vi "zmq_req LabVIEW client.vi"() -> ()   [LabVIEW 2019]
uses:
  <vilib>/addons/zeromq/socket_type.ctl
  <vilib>/addons/zeromq/zmq_context.lvclass
  <vilib>/addons/zeromq/zeromq.lvlib
  <vilib>/addons/zeromq/zmq_socket.lvclass
  erx-demo/eRX 802.15.4/Performance measure context.ctl
panel:
  out "data":string
  out "Measures out":T1 {"Total samples" format="%#_6p"; "Elapsed time" format="%#_6p"; "Samples per second" format="%#_6p"; "Time per sample" format="%#_6p"; "Packets per second" format="%#_6p"; "Last samples per second" format="%#_6p"}
  out "error out":errorcluster
  in  "Stop 2":bool
  in  "Stop":bool
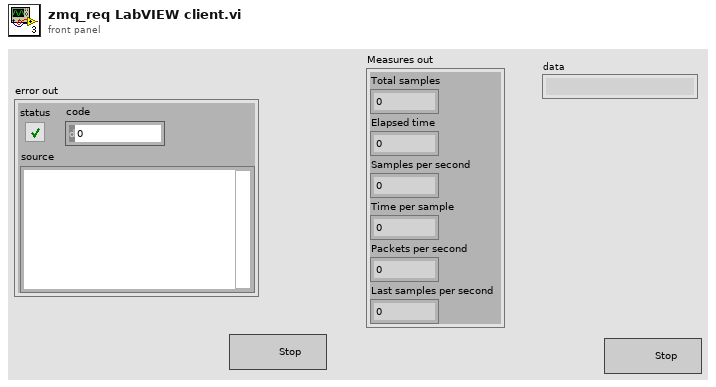
[diagram p1: front panel]
types:
  T1 = cluster{"Total samples":dbl, "Elapsed time":dbl, "Samples per second":dbl, "Time per sample":dbl, "Packets per second":dbl, "Last samples per second":dbl}
  T2 = typedef "zeromq.lvlib/socket_type.ctl" = enum8{"ZMQ_PAIR", "ZMQ_PUB", "ZMQ_SUB", "ZMQ_REQ", "ZMQ_REP", "ZMQ_DEALER", "ZMQ_ROUTER", "ZMQ_PULL", "ZMQ_PUSH", "ZMQ_XPUB", "ZMQ_XSUB"}
  T3 = typedef "Performance measure context.ctl" = cluster{"Seconds decayed":dbl, "Samples decayed":dbl, "Packet count":dbl, "Samples count":dbl, "Timestamp":dbl, "Start time":dbl}
  T4 = enum16{"Standard", "Buffered", "CRLF", "Immediate"}
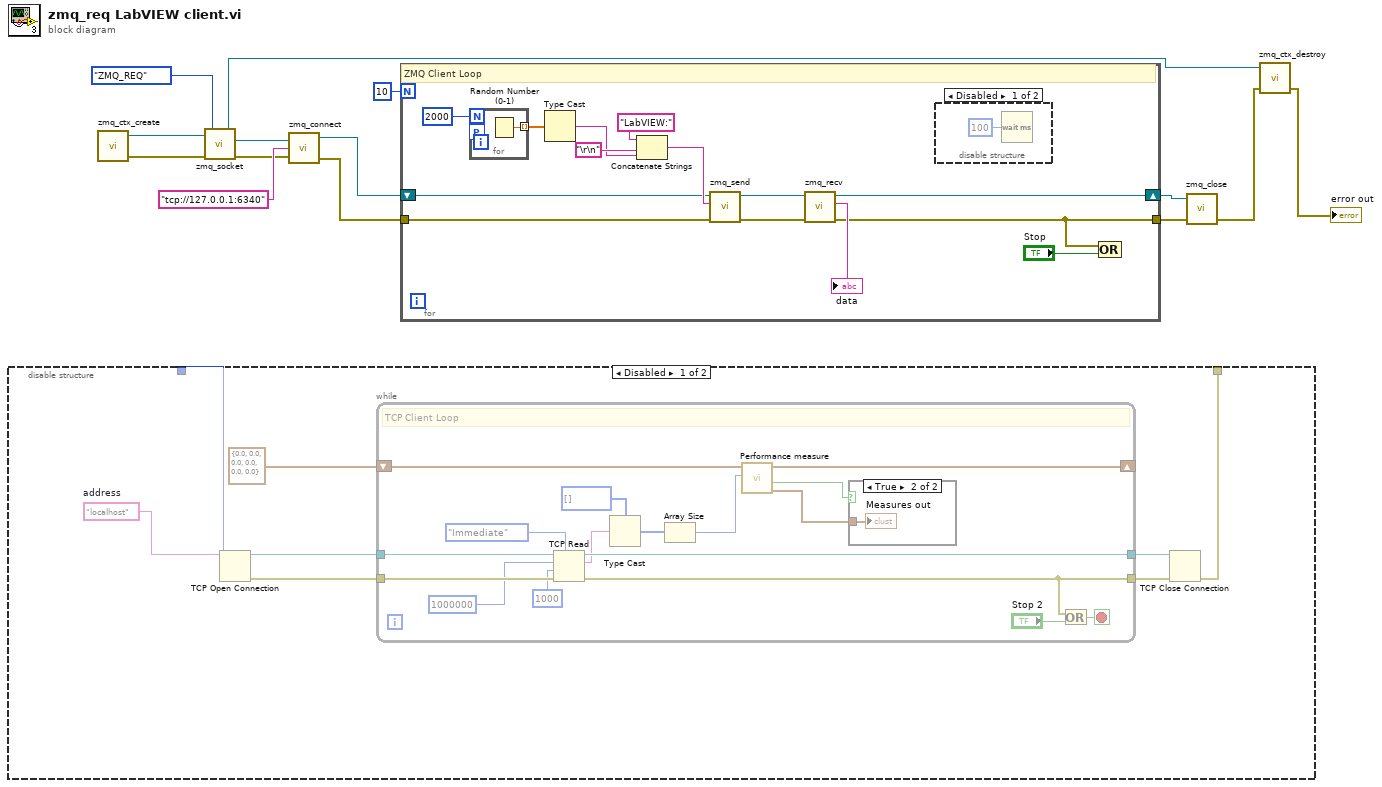
[diagram p0: block diagram]
diagram:
  n1 = disable-structure shown="Disabled" {
    disable-tunnel: [w19 _] -> _
    disable-tunnel: _ -> [w18 _]
    frame Disabled {
      w20 = "localhost"  # address
      n2 = TCP Open Connection(address=w20, remote port or service name=w18) -> (connection ID=w22:refnum<k5>, error out=w21:errorcluster)  [unwired: 3 in]
      n3 = while {
        tunnel: w21 -> [w38]
        tunnel: w22 -> [w39]
        tunnel: [w33] -> w17
        tunnel: [w32] -> w16
        shift-right: [w26] -> _
        shift-left: T3 {"Seconds decayed"=0.0, "Samples decayed"=0.0, "Packet count"=0.0, "Samples count"=0.0, "Timestamp"=0.0, "Start time"=0.0} ("Context out") -> [w25]
        stop <- w36 stop-if-true
        # "TCP Client Loop"
        n4 = TCP Read(connection ID=w39, bytes to read=1000000, error in (no error)=w38, 7:T4."Immediate" ("mode (standard)"), 9:1000 ("timeout ms (25000)")) -> (connection ID out=w33:refnum<k5>, data out=w30:string, error out=w32:errorcluster)
        n5 = Type Cast(type=u8[] [], x=w30) -> (*(type *) &x=w28:u8[])
        n6 = Array Size(array=w28) -> (size(s)=w27:i32)
        n7 = call "Performance measure.vi"("Samples processed"=w27, "Context in"=w25) -> ("Measures out"=w24:T1, "Update"=w23:bool, "Context out"=w26:T3)  [unwired: 7 in]
        n8 = case shown="True" w23 {
          tunnel: w24 -> [_ w40]
          frame False {
          }
          frame True {
            "Measures out" <- w40
          }
        }
        n9 = Or(x=w32, y="Stop 2") -> (x .or. y?=w36:bool)
      }
      n10 = TCP Close Connection(connection ID=w17, error in (no error)=w16) -> (error out=w19:errorcluster)  [unwired: 1 in, 1 out]
    }
    frame Enabled {
    }
  }
  n11 = call <vilib>:"zmq_ctx_create.vi"() -> ("error out"=w14:errorcluster, "context out"=w13:refnum<class "zmq_context.lvclass">)  [unwired: 4 in]
  n12 = call <vilib>:"zmq_socket.vi"("error in"=w14, "socket type"=socket_type."ZMQ_REQ", "context in"=w13) -> ("error out"=w2:errorcluster, "socket out"=w5:refnum<class "zmq_socket.lvclass">, "context out"=w9:refnum<class "zmq_context.lvclass">)  [unwired: 2 in]
  n13 = call <vilib>:"zmq_connect.vi"("error in"=w2, "endpoint"="tcp://127.0.0.1:6340", "socket in"=w5) -> ("error out"=w1:errorcluster, "socket out"=w3:refnum<class "zmq_socket.lvclass">)  [unwired: 1 in]
  n14 = for {
    N: 10 -> [_]
    tunnel: [w44] -> w11
    tunnel: w1 -> [w41]
    shift-right: [w43] -> w10
    shift-left: w3 -> [w42]
    # "ZMQ Client Loop"
    n15 = for {
      N: 2000 ("# of Points") -> [_]
      tunnel: [w56] -> w52 mode=indexing
      workers-P: _ -> [_]
      n16 = Random Number (0-1)() -> (number: 0 to 1=w56:dbl)
    }
    n17 = Type Cast(x=w52) -> (*(type *) &x=w48:string)  [unwired: 1 out]
    n18 = Concatenate Strings("LabVIEW:" ("data"), "\r\n", w48) -> (w47:string)
    n19 = call <vilib>:"zmq_send.vi"("error in"=w41, "data"=w47, "socket in"=w42) -> ("error out"=w45:errorcluster, "socket out"=w46:refnum<class "zmq_socket.lvclass">)  [unwired: 4 in]
    n20 = call <vilib>:"zmq_recv.vi"("error in"=w45, "socket in"=w46) -> ("error out"=w44:errorcluster, "data"=→"data":string, "socket out"=w43:refnum<class "zmq_socket.lvclass">)  [unwired: 3 in, 2 out]
    n21 = disable-structure shown="Disabled" {
      frame Disabled {
        n22 = Wait (ms)(milliseconds to wait=u32 100) -> ()  [unwired: 1 out]
      }
      frame Enabled {
      }
    }
    n23 = Compound Arithmetic op=OR(w44, "Stop") -> ()  [unwired: 1 out]
  }
  n24 = call <vilib>:"zmq_close.vi"("error in"=w11, "socket"=w10) -> ("error out"=w8:errorcluster)  [unwired: 3 in]
  n25 = call <vilib>:"zmq_ctx_destroy.vi"("error in"=w8, "context in"=w9) -> ("error out"=→"error out":errorcluster)  [unwired: 3 in]
